vi "TexttoMercury.vi"() -> ()   [LabVIEW 2015]
uses:
  <instrlib>/Mercury iXX/Public/Libraries/Temperature.lvlib
  <instrlib>/Mercury iXX/Mercury iXX.lvlib
  <instrlib>/Mercury iXX/Public/Controls/Comms Transport Layer.ctl
  <instrlib>/Mercury iXX/Private/Controls/Query Dynamic Reference.ctl
  <instrlib>/Mercury iXX/Public/Controls/Mercury Reference.ctl
  <instrlib>/Mercury iXX/Public/Controls/Unit String.ctl
panel:
  in  "Unit":T1
  out "error out":errorcluster
  out "Mercury Reference Out":T2
  in  "error in":errorcluster
  in  "Mercury Reference In":T2
  out "Data Dsiplay":dbl[][](array[numeric])
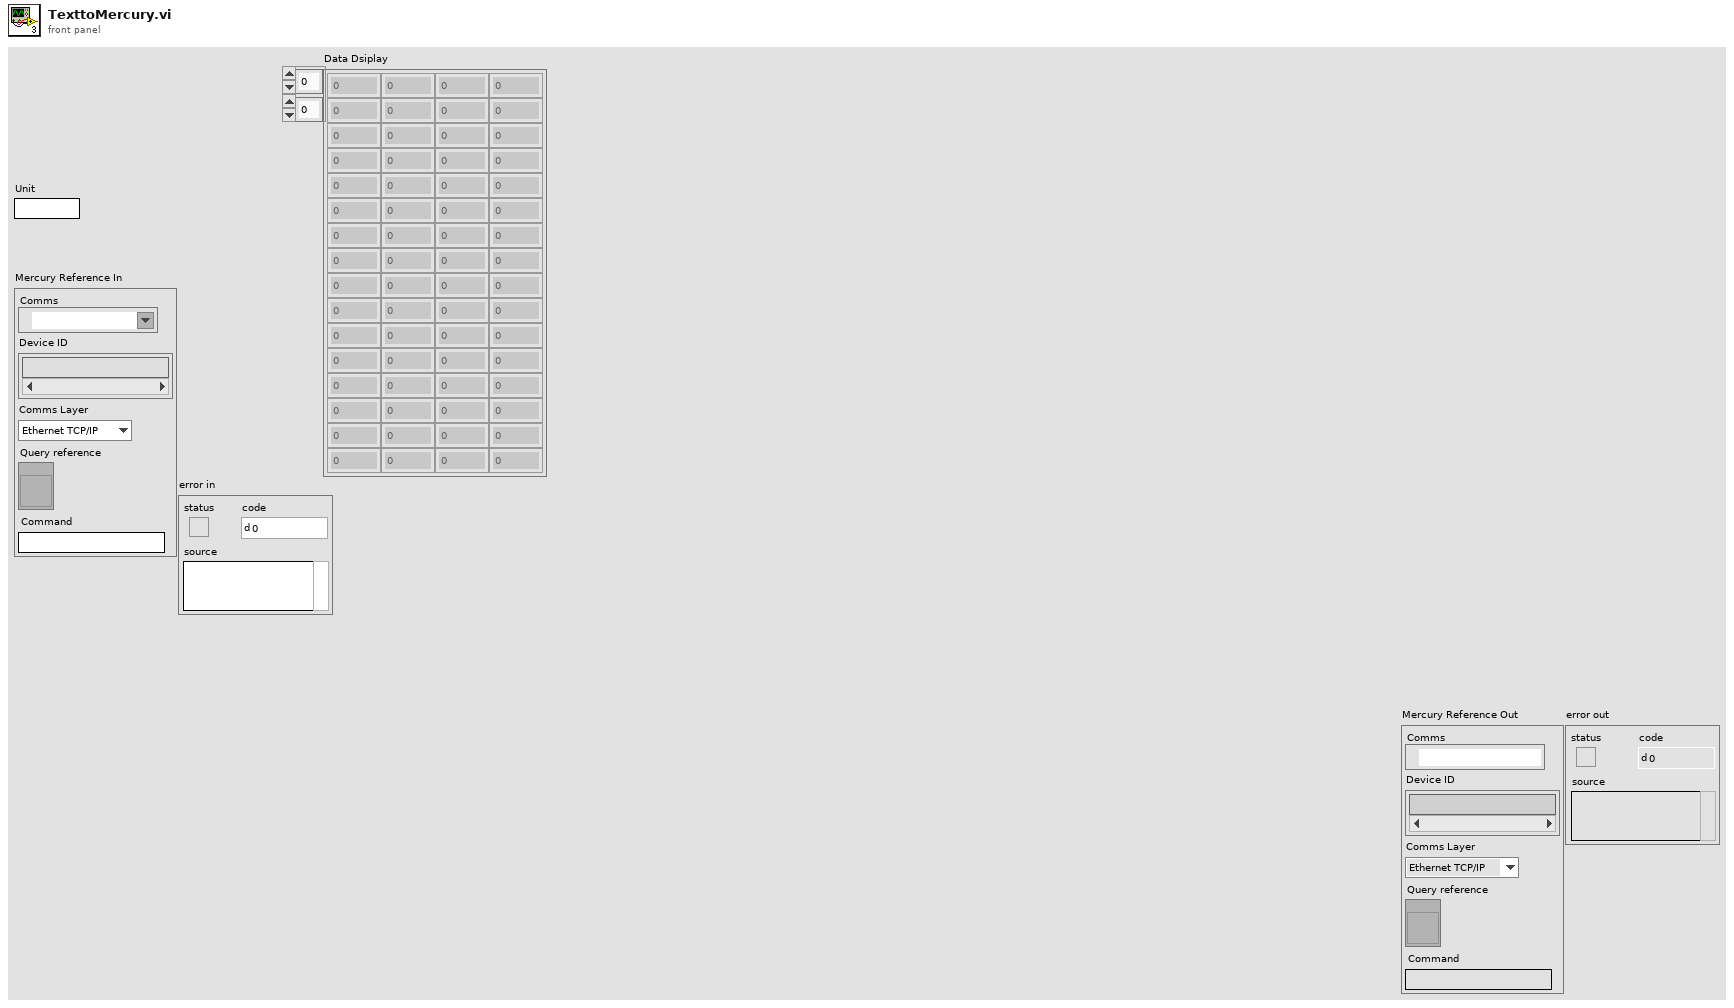
[diagram p1: front panel]
types:
  T1 = typedef "Mercury iXX.lvlib/Unit String.ctl" = string
  T2 = typedef "Mercury iXX.lvlib/Mercury Reference.ctl" = cluster{"Comms":refnum<visa-resource-name>, "Device ID":string[], "Comms Layer":T3, "Command":string, "Query reference":T4}
  T3 = typedef "Mercury iXX.lvlib/Comms Transport Layer.ctl" = enum16{"Ethernet TCP/IP", "USB", "ISOBus - RS-232", "GPIB"}
  T4 = typedef "Mercury iXX.lvlib/Query Dynamic Reference.ctl" = refnum<vi>
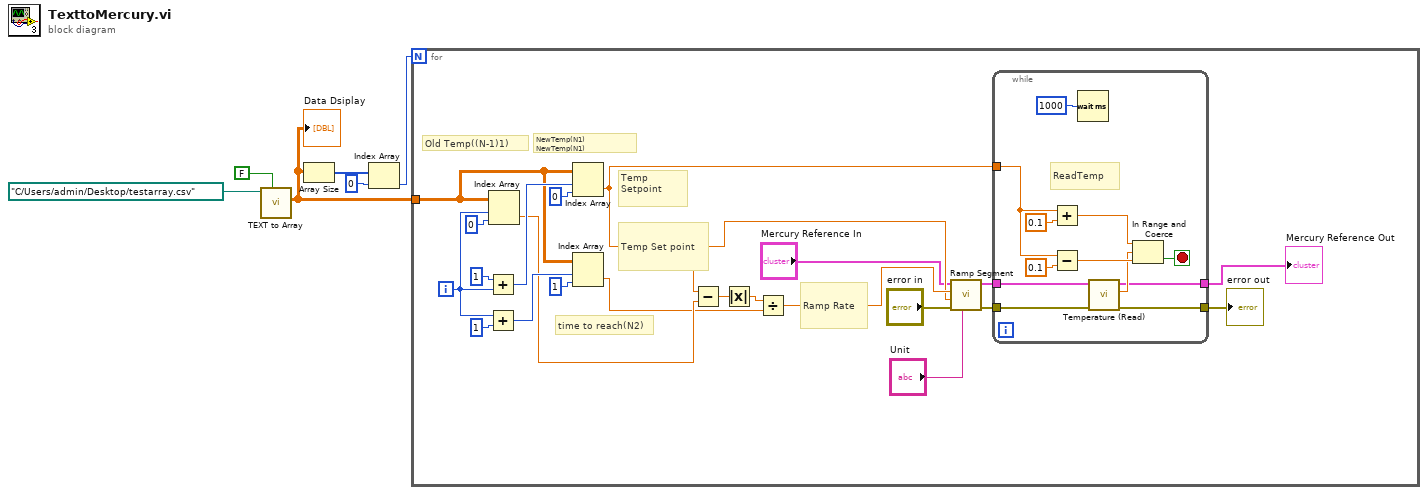
[diagram p0: block diagram]
diagram:
  n1 = call <userlib>:"TEXT to Array.vi"("My File has Row Headers"=FALSE, "Spreadsheet path (.csv)"=path "C:/Users/admin/Desktop/testarray.csv") -> ("Data Dsiplay"=w2:dbl[][])  [unwired: 8 in, 1 out]
  "Data Dsiplay" <- w2
  n2 = Array Size(array=w2) -> (size(s)=w4:i32[])
  n3 = Index Array(array=w4, index=0) -> (element=w1:i32)
  n4 = for {
    N: w1 -> [_]
    tunnel: w2 -> [w21]
    i -> [w16]
    # "Temp Set point"
    # "Ramp Rate"
    # "Temp Setpoint"
    # "time to reach(N2)"
    # "Old Temp((N-1)1)"
    # "NewTemp(N1) NewTemp(N1)"
    n5 = Add(x=1, y=w16) -> (x+y=w26:i32)
    n6 = Add(x=w16, y=1) -> (x+y=w23:i32)
    n7 = Index Array(array=w21, index (row)=w16, index (col)=0) -> (element=w19:dbl)
    n8 = Index Array(array=w21, index (row)=w26, index (col)=0) -> (element=w14:dbl)
    n9 = Index Array(array=w21, index (row)=w23, index (col)=1) -> (element=w18:dbl)
    n10 = Subtract(x=w14, y=w19) -> (x-y=w20:dbl)
    n11 = Absolute Value(x=w20) -> (abs(x)=w17:dbl)
    n12 = Divide(x=w17, y=w18) -> (x/y=w15:dbl)
    n13 = call <userlib>:"Ramp Segment.vi"("Unit"="Unit", "error in"="error in", "Temperature setpoint"=w14, "Ramp rate"=w15, "Mercury Reference In"="Mercury Reference In") -> ("error out"=w10:errorcluster, "Mercury Reference Out"=w12:T2)  [unwired: 5 in]
    n14 = while {
      tunnel: w14 -> [w38]
      tunnel: w12 -> [w33]
      tunnel: w10 -> [w31]
      tunnel: [w30] -> w8
      tunnel: [w29] -> w9
      stop <- w39 stop-if-true
      # "ReadTemp"
      n15 = Add(x=w38, y=0.1) -> (x+y=w34:dbl)
      n16 = Subtract(x=w38, y=0.1) -> (x-y=w35:dbl)
      n17 = Wait (ms)(milliseconds to wait=1000) -> ()  [unwired: 1 out]
      n18 = call <instrlib>:"Temperature (Read).vi"("error in"=w31, "Mercury Reference In"=w33) -> ("error out"=w30:errorcluster, "Temperature"=w32:dbl, "Mercury Reference Out"=w29:T2)  [unwired: 5 in, 2 out]
      n19 = In Range and Coerce(upper limit=w34, x=w32, lower limit=w35) -> (In Range?=w39:bool)  [unwired: 1 out]
    }
    "Mercury Reference Out" <- w9
    "error out" <- w8
  }
